vi "SetCoeffOrder.vi"(8 "error in (no error)":errorcluster, 10 "Order":string, 11 "CoeFile in":refnum<class "CoeFile.lvclass">) -> (0 "error out":errorcluster, 3 "CoeFile out":refnum<class "CoeFile.lvclass">)   [LabVIEW 2013, in "CoeFile.lvclass"]
uses:
  CoeFile.lvclass
  CoeFile.lvclass/CoeFile.ctl
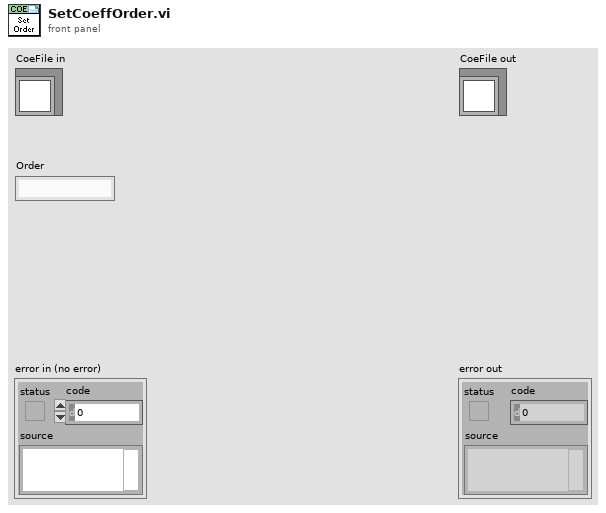
[diagram p1: front panel]
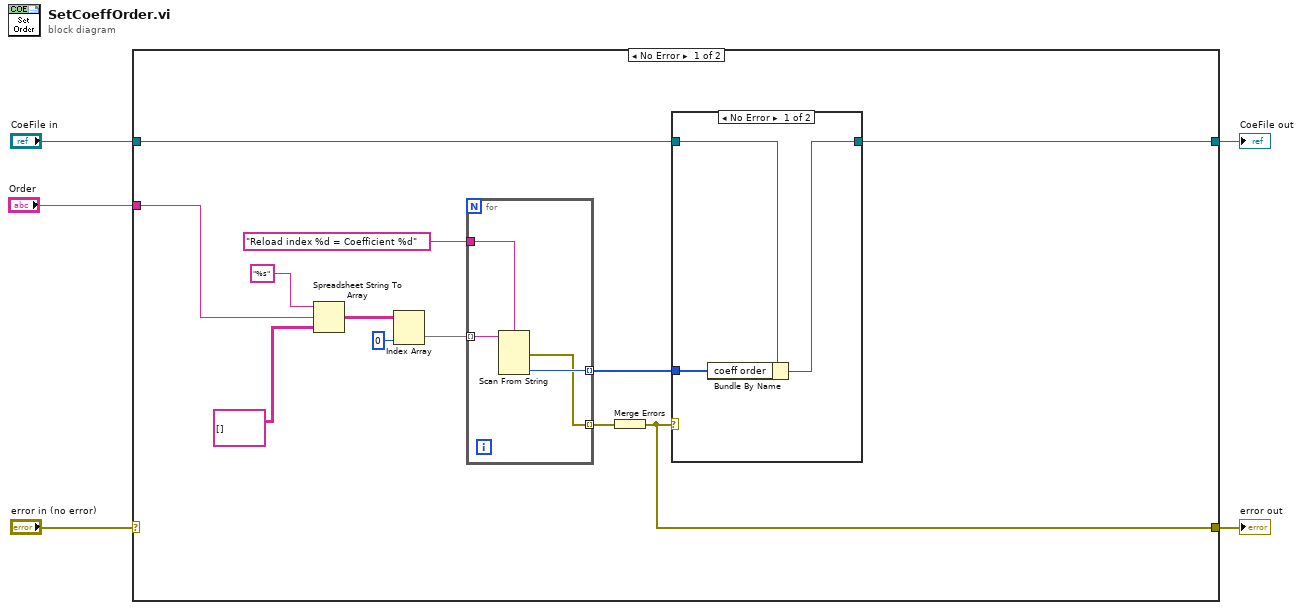
[diagram p0: block diagram]
diagram:
  n1 = case shown="No Error" "error in (no error)" {
    selector: "error in (no error)" -> [_ w27]
    tunnel: [w6 w27] -> w4
    tunnel: [w7 w26] -> w2
    tunnel: "CoeFile in" -> [w10 w26]
    tunnel: "Order" -> [w13 _]
    frame No Error {
      n2 = Spreadsheet String To Array(format string="%s", spreadsheet string=w13, array type (2D Dbl)=string[][] []) -> (array=w14:string[][])  [unwired: 1 in]
      n3 = Index Array(array=w14, index (col)=0 ("disabled index (col)")) -> (element=w12:string[])  [unwired: 1 in]
      n4 = for {
        tunnel: w12 -> [w25] mode=indexing
        tunnel: "Reload index %d = Coefficient %d" -> [w24]
        tunnel: [w23] -> w8 mode=indexing
        tunnel: [w22] -> w9 mode=indexing
        n5 = Scan From String(format string=w24, input string=w25) -> (error out=w22:errorcluster, output 2=w23:i32)  [unwired: 5 in, 2 out]
      }
      n6 = Merge Errors(w9) -> (w6:errorcluster)
      n7 = case shown="No Error" w6 {
        tunnel: w10 -> [w20 w21]
        tunnel: w8 -> [w19 _]
        tunnel: [w18 w21] -> w7
        frame No Error {
          n8 = Bundle By Name(cluster=w20, "coeff order"=w19) -> (w18:refnum<class "CoeFile.lvclass">)
        }
        frame Error {
        }
      }
    }
    frame Error {
    }
  }
  "error out" <- w4
  "CoeFile out" <- w2
